vi "DPOreadFrequency.vi"(3 "错误输入（无错误）":errorcluster, 5 "VISA资源名称":refnum<visa-resource-name>) -> (0 "错误输出":errorcluster, 1 "重复频率":dbl, 2 "VISA资源名称输出":refnum<visa-resource-name>)   [LabVIEW 2012]
panel:
  out "data out":string
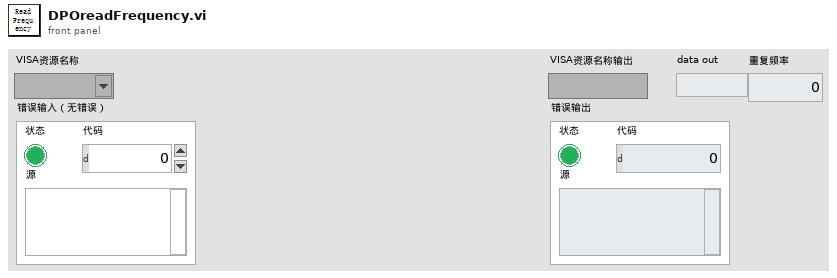
[diagram p1: front panel]
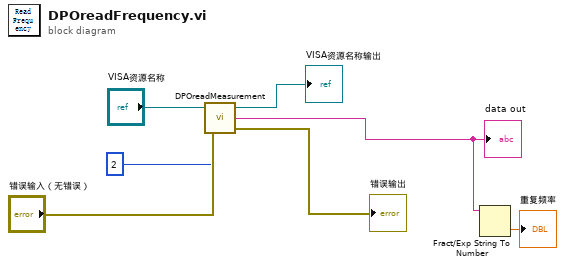
[diagram p0: block diagram]
diagram:
  n1 = call "DPOreadMeasurement.vi"("错误输入（无错误）"="错误输入（无错误）", "通道"=u8 2, "VISA资源名称"="VISA资源名称") -> ("错误输出"=→"错误输出":errorcluster, "data out"=w2:string, "VISA资源名称输出"=→"VISA资源名称输出":refnum<visa-resource-name>)
  "data out" <- w2
  n2 = Fract/Exp String To Number(string=w2) -> (number=→"重复频率":dbl)  [unwired: 3 in, 1 out]
